vi "Load Log Man.vi"(8 "error in (no error)":errorcluster, 10 "Log Config Path":path, 11 "Caller Actor in":refnum<class "Actor.lvclass">) -> (0 "error out":errorcluster, 3 "Caller Actor out":refnum<class "Actor.lvclass">)   [LabVIEW 2020, in "Logging.lvlib" / "Logger Mananger.lvclass"]
uses:
  Logger Mananger.lvclass
  <vilib>/ActorFramework/Actor/Actor.lvclass
  C:/Program Files (x86)/National Instruments/LabVIEW 2020/vi.lib/ActorFramework/Actor/Actor.lvclass
  Logger Mananger.lvclass/Logger Mananger.ctl
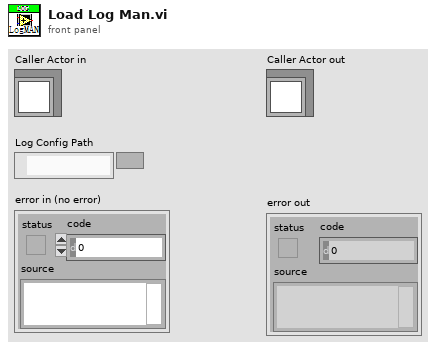
[diagram p1: front panel]
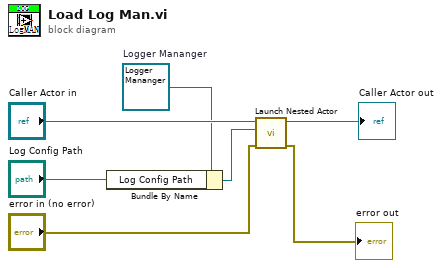
[diagram p0: block diagram]
diagram:
  w3 = refnum<class "Logger Mananger.lvclass"> refnum  # Logger Mananger
  n1 = Bundle By Name(cluster=w3, "Log Config Path"="Log Config Path") -> (w2:refnum<class "Logger Mananger.lvclass">)
  n2 = call <vilib>:"Launch Nested Actor.vi"("error in (no error)"="error in (no error)", "Nested Actor"=w2, "Caller Actor in"="Caller Actor in") -> ("error out"=→"error out":errorcluster, "Caller Actor out"=→"Caller Actor out":refnum<class "Actor.lvclass">)  [unwired: 6 in, 1 out]
